vi "BRig_RT__Case_Exp__State_initTrial4.vi"(6 "input_Recording":bool, 8 "input_FPGA_count2ms":dbl, 10 "input_dataTrial":u16[][](array[numeric])) -> (0 "output_Solenoid_nTotal":u32, 2 "output_dataTrial":u16[][](array[numeric]))   [LabVIEW 2014]
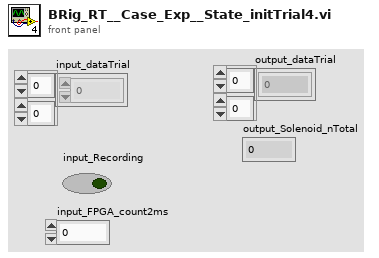
[diagram p1: front panel]
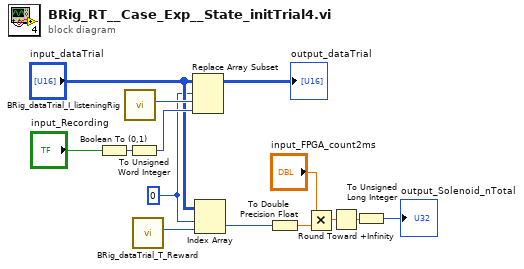
[diagram p0: block diagram]
diagram:
  w1 = 0
  n1 = Boolean To (0,1)(Boolean="input_Recording") -> (0, 1=w14:i16)
  n2 = call "BRig_dataTrial_I_listeningRig.vi"() -> ("output_I_listeningRig"=w12:i32)  [unwired: 11 in]
  n3 = To Unsigned Word Integer(number=w14) -> (unsigned 16bit integer=w11:u16)
  n4 = call "BRig_dataTrial_T_Reward.vi"() -> ("output_T_Reward"=w13:i32)  [unwired: 11 in]
  n5 = Replace Array Subset(array="input_dataTrial", new element=w11, index (row)=w1, index (col)=w12) -> (→"output_dataTrial":u16[][])
  n6 = Index Array(array="input_dataTrial", index (row)=w1, index (col)=w13) -> (element=w4:u16)
  n7 = To Double Precision Float(number=w4) -> (double precision float=w5:dbl)
  n8 = Multiply(x="input_FPGA_count2ms", y=w5) -> (x*y=w6:dbl)
  n9 = Round Toward +Infinity(x=w6) -> (ceil(x): smallest int >= x=w7:dbl)
  n10 = To Unsigned Long Integer(number=w7) -> (unsigned 32bit integer=→"output_Solenoid_nTotal":u32)
